vi "DS18B20_Convert Raw Temp.vi"(9 "Scratchpad Data":u8[](array[numeric])=[0, 0, 0, 0, 0, 0, 0, 0, 0]) -> (1 "Temp (F)":sgl, 2 "Temp rounded (C)":dbl, 3 "Temp (C)":sgl)   [LabVIEW 2020]
panel:
  out "MSB":u8 format="%.0x"
  out "LSB":u8 format="%.0x"
  # "Perform the temperature conversion for DS18B20\n- takes the scratchpad data from the device \n- calculates temperature in C and F"
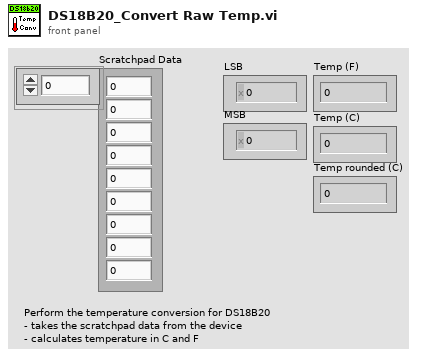
[diagram p1: front panel]
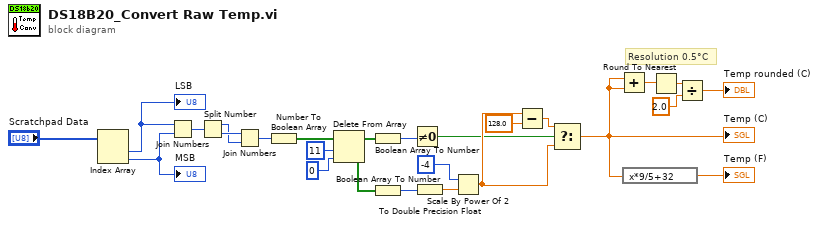
[diagram p0: block diagram]
diagram:
  # "Resolution 0.5°C"
  n1 = Index Array(array="Scratchpad Data") -> (element #1=w8:u8, element #2=w9:u8)  [unwired: 2 in]
  "LSB" <- w8
  "MSB" <- w9
  n2 = Join Numbers(hi=w8, lo=w9) -> ((hi.lo)=w11:u16)
  n3 = Split Number(x=w11) -> (hi(x)=w6:u8, lo(x)=w7:u8)
  n4 = Join Numbers(hi=w7, lo=w6) -> ((hi.lo)=w24:u16)
  n5 = Number To Boolean Array(number=w24) -> (Boolean array=w23:bool[])
  n6 = Delete From Array(array=w23, length=11, index=0) -> (deleted portion=w20:bool[], array with subset deleted=w15:bool[])
  n7 = Boolean Array To Number(Boolean array=w15) -> (number=w14:u8)
  n8 = Boolean Array To Number(Boolean array=w20) -> (number=w17:u16)
  n9 = Not Equal To 0?(x=w14) -> (x != 0?=w13:bool)
  n10 = To Double Precision Float(number=w17) -> (double precision float=w18:dbl)
  n11 = Scale By Power Of 2(n=-4, x=w18) -> (x*2^n=w16:dbl)
  n12 = Subtract(x=w16, y=128.0 ("x")) -> (x-y=w26:dbl)
  n13 = Select(t=w26, s=w13, f=w16) -> (s? t:f=w5:dbl)
  "Temp (C)" <- w5
  n14 = Add(x=w5, y=w5) -> (x+y=w4:dbl)
  n15 = expression code="x*9/5+32"(w5) -> (→"Temp (F)":dbl)
  n16 = Round To Nearest(number=w4) -> (nearest integer value=w3:dbl)
  n17 = Divide(x=w3, y=2.0) -> (x/y=→"Temp rounded (C)":dbl)
